vi "F Dwf Analog In Trigger Position Info.vi"(7 "pnSteps":dbl, 8 "error in (no error)":errorcluster, 9 "psecMax":dbl, 10 "psecMin":dbl, 11 "hdwf":i32) -> (0 "error out":errorcluster, 1 "psecMax out":dbl, 2 "psecMin out":dbl, 3 "function return":i32, 5 "pnSteps out":dbl)   [LabVIEW 2019, in "Olasdwf.lvlib"]
doc: "DWFAPI int FDwfAnalogInTriggerPositionInfo(HDWF hdwf, double *psecMin, double *psecMax, double *pnSteps);"
uses:
  Olasdwf.lvlib
  Windows/System32/dwf.dll
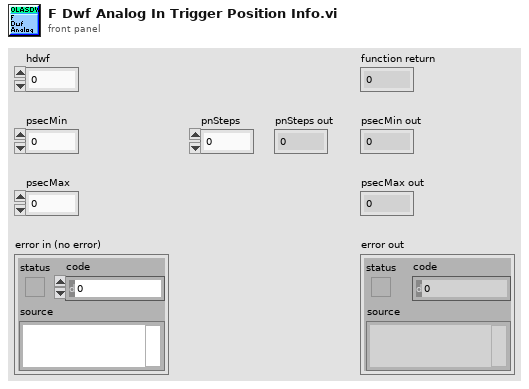
[diagram p1: front panel]
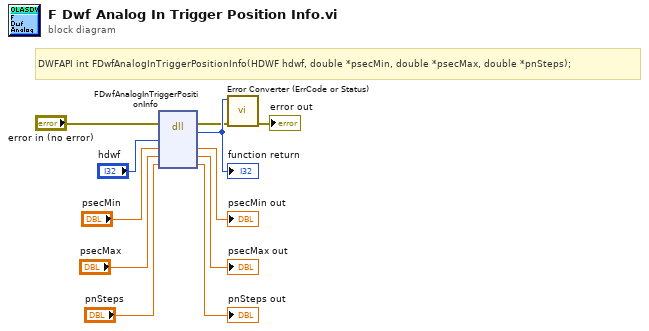
[diagram p0: block diagram]
diagram:
  # "DWFAPI int FDwfAnalogInTriggerPositionInfo(HDWF hdwf, double *psecMin, double *psecMax, double *pnSteps);"
  n1 = dll-call lib="C:/Windows/System32/dwf.*" fn="FDwfAnalogInTriggerPositionInfo"(error in="error in (no error)", "hdwf"="hdwf", "psecMin"="psecMin", "psecMax"="psecMax", "pnSteps"="pnSteps") -> (error out=w2:errorcluster, w11:i32, "psecMin"=→"psecMin out":dbl, "psecMax"=→"psecMax out":dbl, "pnSteps"=→"pnSteps out":dbl)  [unwired: 3 in, 1 out]
  "function return" <- w11
  n2 = call "Error Converter (ErrCode or Status).vi"("error in (no error)"=w2, "error code"=w11) -> ("error out"=→"error out":errorcluster)  [unwired: 9 in]
